vi "EXCEL report.vi"(7 "Report state":T1=enum."Close report", 8 "error in":errorcluster, 10 "Data in":variant) -> (0 "error out":errorcluster, 2 "Data out":variant)   [LabVIEW 2015, in "Report.lvlib"]
uses:
  Report.lvlib
  TypeDefs/Report state.ctl
  <vilib>/Utility/NIReport.llb/NI_report.lvclass
  <vilib>/Utility/NIReport.llb/Append Numeric Table to Report (wrap).vi
  <vilib>/Utility/NIReport.llb/NI_ReportGenerationCore.lvlib
  <vilib>/Utility/NIReport.llb/Excel/NI_Excel.lvclass
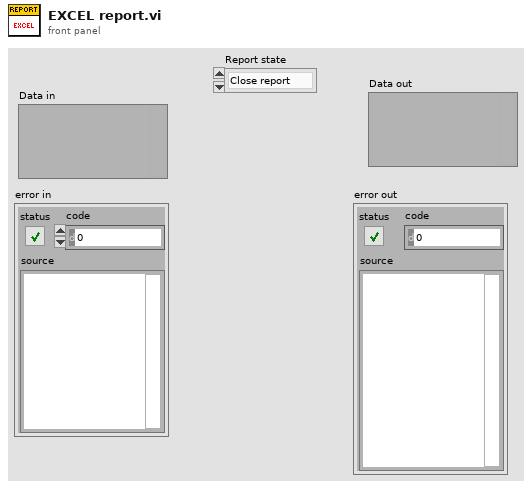
[diagram p1: front panel]
types:
  T1 = typedef "Report.lvlib/Report state.ctl" = enum16{"Create report", "Save data", "Save report", "Available printers", "Print report", "Close report"}
  T2 = enum16{"Standard Report", "HTML", "Word", "Excel"}
  T3 = enum16{"maximized", "minimized", "normal", "no change"}
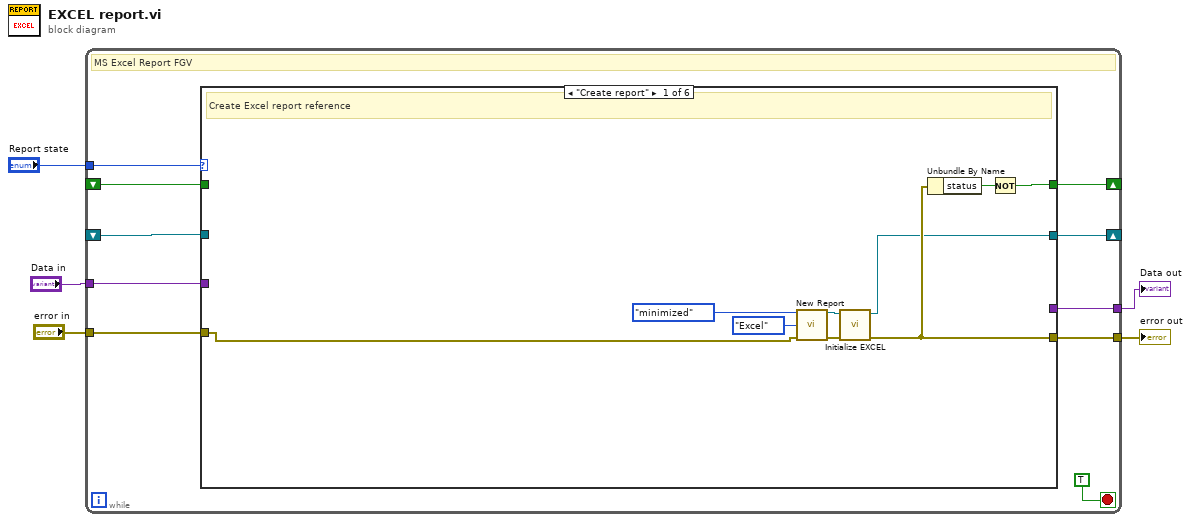
[diagram p0: block diagram]
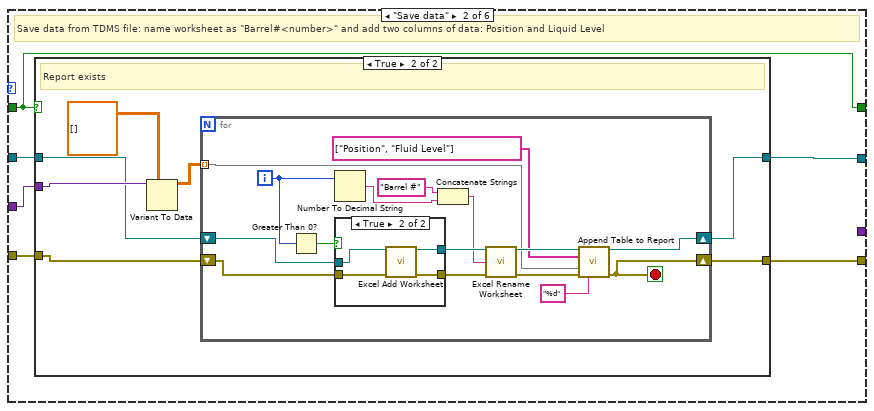
[diagram p2: hidden frame]
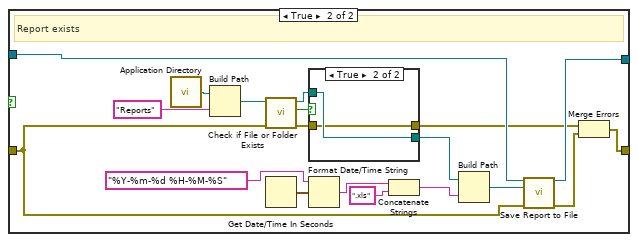
[diagram p6: hidden frame]
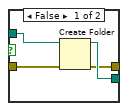
[diagram p7: hidden frame]
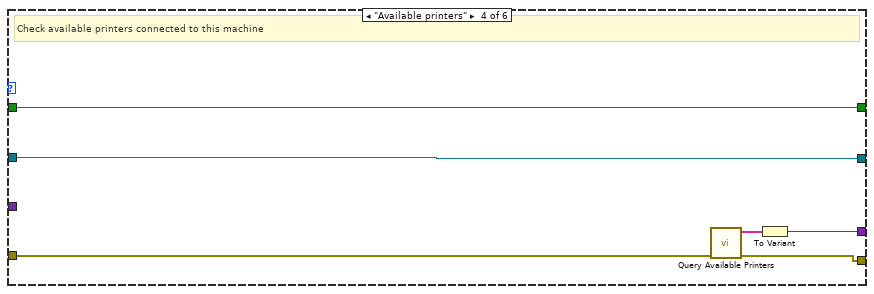
[diagram p8: hidden frame]
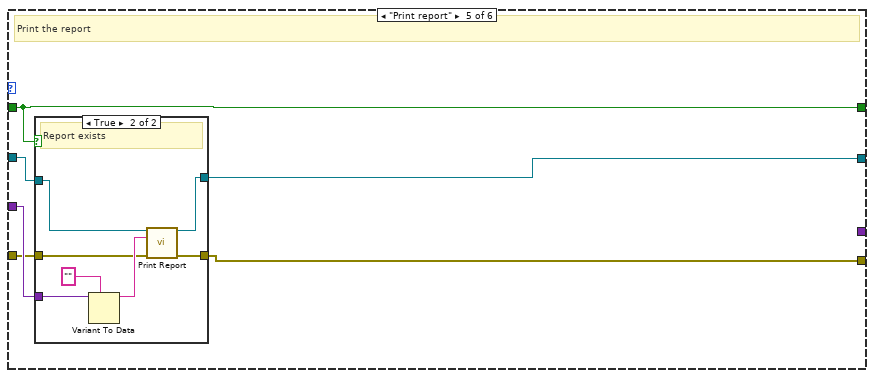
[diagram p9: hidden frame]
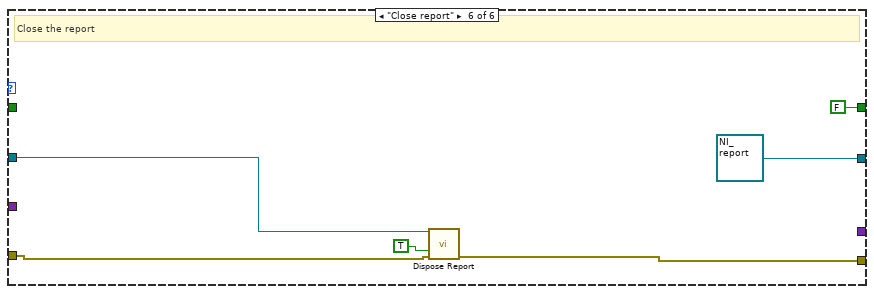
[diagram p11: hidden frame]
diagram:
  n1 = while {
    tunnel: "Report state" -> [w13]
    tunnel: "Data in" -> [w14]
    tunnel: "error in" -> [w12]
    tunnel: [w11] -> w2
    tunnel: [w10] -> w1
    shift-right: [w8] -> _
    shift-left: _ -> [w9]
    shift-right: [w7] -> _
    shift-left: _ -> [w6]
    stop <- TRUE stop-if-true
    # "MS Excel Report FGV"
    n2 = case shown="\"Create report\"" w13 {
      tunnel: w14 -> [_ w30 _ _ w105 _]
      tunnel: w12 -> [w20 w27 w64 w97 w102 w115]
      tunnel: [_ _ _ w98 _ _] -> w11
      tunnel: [w19 w29 w66 w96 w104 w119] -> w10
      tunnel: w9 -> [_ w28 w65 w95 w103 _]
      tunnel: [w17 w28 w65 w95 w103 FALSE] -> w8
      tunnel: [w16 w25 w62 w94 w100 refnum<class "NI_report.lvclass"> refnum ("Report ID")] -> w7
      tunnel: w6 -> [_ w26 w63 w94 w101 w117]
      frame "Create report" {
        # "Create Excel report reference"
        n3 = call <vilib>:"New Report.vi"("window state (normal)"=T3."minimized", "report type"=T2."Excel", "error in (no error)"=w20) -> ("report out"=w22:refnum<class "NI_report.lvclass">, "error out"=w21:errorcluster)  [unwired: 11 in]
        n4 = call "Initialize EXCEL.vi"("error in (no error)"=w21, "NI_report in"=w22) -> ("error out"=w19:errorcluster, "NI_report out"=w16:refnum<class "NI_report.lvclass">)  [unwired: 8 in]
        n5 = Unbundle By Name(w19) -> ("status"=w18:bool)
        n6 = Not(x=w18) -> (.not. x?=w17:bool)
      }
      frame "Save data" {
        # "Save data from TDMS file: name worksheet as \"Barrel#<number>\" and add two columns of data: Position and Liquid Level"
        n7 = case shown="True" w28 {
          tunnel: w30 -> [_ w39]
          tunnel: [w32 w36] -> w29
          tunnel: w27 -> [w32 w34]
          tunnel: w26 -> [w31 w35]
          tunnel: [w31 w33] -> w25
          frame False {
            # "Report not created"
          }
          frame True {
            # "Report exists"
            n8 = Variant To Data(type=dbl[][][] [], Variant=w39) -> (data=w37:dbl[][][])  [unwired: 1 in, 1 out]
            n9 = for {
              tunnel: w37 -> [w44] mode=indexing
              shift-right: [w40] -> w36
              shift-left: w34 -> [w50]
              shift-right: [w45] -> w33
              shift-left: w35 -> [w51]
              i -> [w52]
              stop <- w40 stop-if-true
              n10 = Greater Than 0?(x=w52) -> (x > 0?=w53:bool)
              n11 = Number To Decimal String(number=w52) -> (decimal integer string=w54:string)  [unwired: 1 in]
              n12 = case shown="True" w53 {
                tunnel: w51 -> [w57 w61]
                tunnel: w50 -> [w56 w60]
                tunnel: [w57 w59] -> w49
                tunnel: [w56 w58] -> w48
                frame False {
                }
                frame True {
                  n13 = call <vilib>:"Excel Add Worksheet.vi"("report in"=w61, "error in (no error)"=w60) -> ("report out"=w59:refnum<class "NI_report.lvclass">, "error out"=w58:errorcluster)  [unwired: 12 in]
                }
              }
              n14 = Concatenate Strings("Barrel #", w54) -> (w43:string)
              n15 = call <vilib>:"Excel Rename Worksheet.vi"("report in"=w49, "worksheet name (\"\")"=w43, "error in (no error)"=w48) -> ("report out"=w47:refnum<class "NI_report.lvclass">, "error out"=w46:errorcluster)  [unwired: 11 in]
              n16 = call-poly <vilib>:"Append Table to Report.vi"("report in"=w47, "column headers"=string[] ["Position", "Fluid Level"], "numerical data"=w44, "error in (no error)"=w46, "format string (%.3f)"="%d") -> ("report out"=w45:refnum<class "NI_report.lvclass">, "error out"=w40:errorcluster)  [unwired: 7 in, 2 out]
            }
          }
        }
      }
      frame "Save report" {
        # "Save Excel report on HDD"
        n17 = case shown="False" w65 {
          tunnel: [w68 w69] -> w66
          tunnel: w64 -> [w68 w74]
          tunnel: w63 -> [w67 w73]
          tunnel: [w67 w72] -> w62
          frame False {
            # "Report not created"
          }
          frame True {
            # "Report exists"
            n18 = call <vilib>:"Application Directory.vi"() -> ("Application Directory"=w81:path)
            n19 = Build Path(base path=w81, name or relative path="Reports") -> (appended path=w79:path)
            n20 = call <vilib>:"Check if File or Folder Exists.vi"("error in (no error)"=w74, "path"=w79) -> ("error out"=w75:errorcluster, "file or folder exists?"=w78:bool, "dup path"=w77:path)  [unwired: 7 in]
            n21 = Get Date/Time In Seconds() -> (seconds since 1Jan1904=w86:timestamp)
            n22 = case shown="True" w78 {
              tunnel: w77 -> [w91 w93]
              tunnel: [w90 w93] -> w76
              tunnel: w75 -> [w89 w92]
              tunnel: [w88 w92] -> w71
              frame False {
                n23 = Create Folder(path (use dialog)=w91, error in=w89) -> (created path=w90:path, error out=w88:errorcluster)  [unwired: 1 in, 1 out]
              }
              frame True {
              }
            }
            n24 = Format Date/Time String(time format string (%c)="%Y-%m-%d %H-%M-%S", seconds (now)=w86) -> (date/time string=w84:string)  [unwired: 1 in]
            n25 = Concatenate Strings(w84, ".xls" ("string")) -> (w82:string)
            n26 = Build Path(base path=w76, name or relative path=w82) -> (appended path=w87:path)
            n27 = call-dynamic "Save Report to File.vi"("report in"=w73, "report file path"=w87, "error in (no error)"=w74) -> ("report out"=w72:refnum<class "NI_report.lvclass">, "error out"=w70:errorcluster)  [unwired: 11 in]
            n28 = Merge Errors(w71, w70) -> (w69:errorcluster)
          }
        }
      }
      frame "Available printers" {
        # "Check available printers connected to this machine"
        n29 = call <vilib>:"Query Available Printers.vi"("error in (no error)"=w97) -> ("error out"=w96:errorcluster, "system configured printers"=w99:string[])  [unwired: 8 in, 1 out]
        n30 = To Variant(anything=w99) -> (Variant=w98:variant)
      }
      frame "Print report" {
        # "Print the report"
        n31 = case shown="True" w103 {
          tunnel: w105 -> [_ w114]
          tunnel: [w107 w111] -> w104
          tunnel: w102 -> [w107 w108]
          tunnel: w101 -> [w106 w110]
          tunnel: [w106 w109] -> w100
          frame False {
            # "Report not created"
          }
          frame True {
            # "Report exists"
            n32 = Variant To Data(type="", Variant=w114) -> (data=w112:string)  [unwired: 1 in, 1 out]
            n33 = call-dynamic "Print Report.vi"("report in"=w110, "printer name (default)"=w112, "error in (no error)"=w108) -> ("report out"=w109:refnum<class "NI_report.lvclass">, "error out"=w111:errorcluster)  [unwired: 11 in]
          }
        }
      }
      frame "Close report" {
        # "Close the report"
        n34 = call-dynamic "Dispose Report.vi"("report in"=w117, "save changes? (F)"=TRUE, "error in (no error)"=w115) -> ("error out"=w119:errorcluster)  [unwired: 12 in]
      }
    }
  }
  "error out" <- w1
  "Data out" <- w2
